vi "Simple XOR Cipher.vi"(9 "key (\"\": random)":string, 11 "data in":string) -> (1 "key out":string, 3 "data out":string)   [LabVIEW 2016]
panel:
  # "Copyright © 2006-2017 JKI. All rights reserved.\n\nThis library is provided \"AS IS\" , WITHOUT WARRANTIES OR \nCONDITIONS OF ANY KIND, either express or implied.\n\nJKI -- http://jki.net"
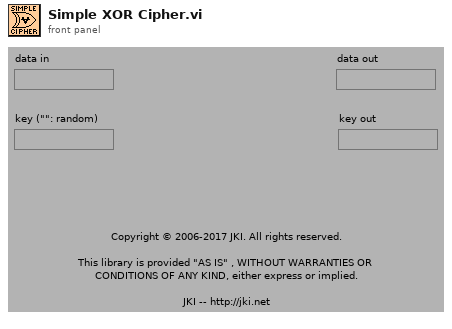
[diagram p1: front panel]
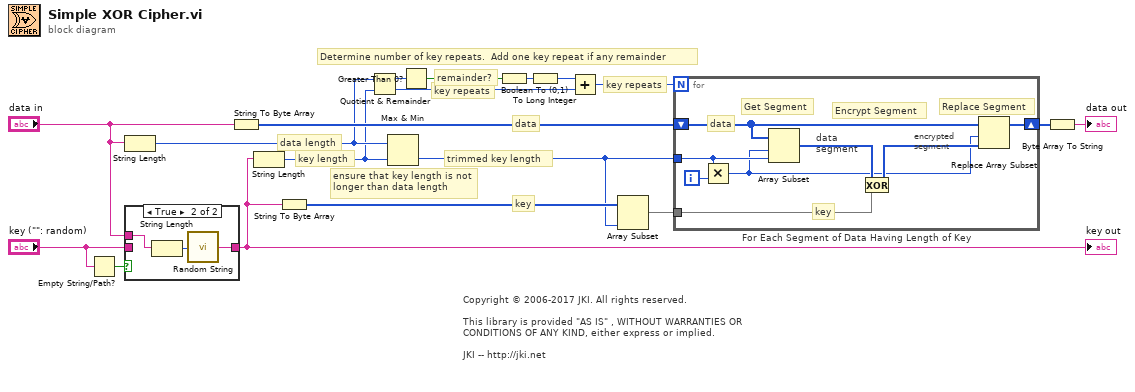
[diagram p0: block diagram]
diagram:
  # "Copyright © 2006-2017 JKI. All rights reserved.\n\nThis library is provided \"AS IS\" , WITHOUT WARRANTIES OR \nCONDITIONS OF ANY KIND, either express or implied.\n\nJKI -- http://jki.net"
  # "key"
  # "data"
  # "Determine number of key repeats.  Add one key repeat if any remainder"
  # "ensure that key length is not longer than data length"
  # "trimmed key length"
  # "data length"
  # "key length"
  # "key repeats"
  # "remainder?"
  # "key repeats"
  n1 = Empty String/Path?(string/path="key (\"\": random)") -> (empty?=w4:bool)
  n2 = String Length(string="data in") -> (length=w14:i32)
  n3 = case shown="True" w4 {
    tunnel: "key (\"\": random)" -> [w19 _]
    tunnel: [w19 w21] -> w2
    tunnel: "data in" -> [_ w20]
    frame False {
    }
    frame True {
      n4 = String Length(string=w20) -> (length=w22:i32)
      n5 = call "Random String.vi"("length"=w22) -> ("random data"=w21:string)  [unwired: 4 in]
    }
  }
  "key out" <- w2
  n6 = String To Byte Array(string="data in") -> (unsigned byte array=w18:u8[])
  n7 = String Length(string=w2) -> (length=w13:i32)
  n8 = String To Byte Array(string=w2) -> (unsigned byte array=w16:u8[])
  n9 = Quotient & Remainder(x=w14, y=w13) -> (x-y*floor(x/y)=w12:i32, floor(x/y)=w9:i32)
  n10 = Max & Min(x=w14, y=w13) -> (min(x,y)=w7:i32)  [unwired: 1 out]
  n11 = Greater Than 0?(x=w12) -> (x > 0?=w11:bool)
  n12 = Boolean To (0,1)(Boolean=w11) -> (0, 1=w10:i16)
  n13 = To Long Integer(number=w10) -> (32bit integer=w5:i32)
  n14 = Add(x=w5, y=w9) -> (x+y=w8:i32)
  n15 = Array Subset(array=w16, length=w7) -> (w6:u8[])  [unwired: 1 in]
  n16 = for "For Each Segment of Data Having Length of Key" {
    N: w8 -> [_]
    shift-right: [w27] -> w17
    shift-left: w18 -> [w28]
    tunnel: w7 -> [w24]
    tunnel: w6 -> [w30]
    i -> [w25]
    # "Replace Segment"
    # "Encrypt Segment"
    # "encrypted segment"
    # "Get Segment"
    # "data segment"
    # "data"
    # "key"
    n17 = Multiply(x=w24, y=w25) -> (x*y=w23:i32)
    n18 = Array Subset(array=w28, index=w23, length=w24) -> (w29:u8[])
    n19 = Exclusive Or(1:w30, 2:w29) -> (0:w26:u8[])
    n20 = Replace Array Subset(array=w28, new element=w26, index=w23) -> (w27:u8[])
  }
  n21 = Byte Array To String(unsigned byte array=w17) -> (string=→"data out":string)
